vi "Read Number of peaks.vi"(8 "error in (no error)":errorcluster, 11 "Micron Optics Driver in":refnum<class "Micron Optics Driver.lvclass">) -> (0 "error out":errorcluster, 2 "Number of peaks":i32=4, 3 "Micron Optics Driver out":refnum<class "Micron Optics Driver.lvclass">)   [LabVIEW 2016, in "Micron Optics Driver.lvclass"]
uses:
  Micron Optics Driver.lvclass
  Micron Optics Driver.lvclass/Micron Optics Driver.ctl
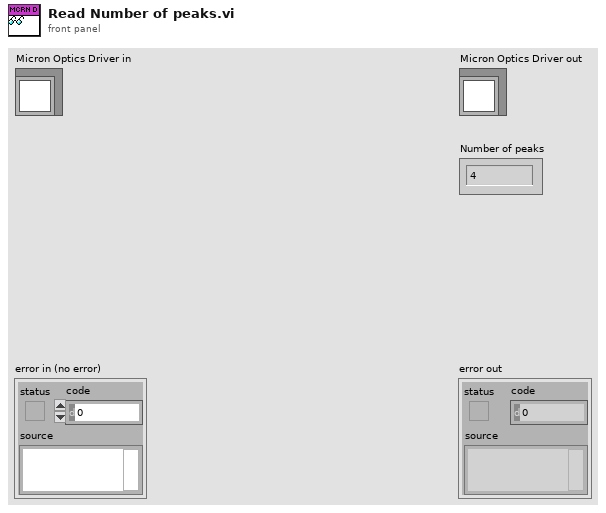
[diagram p1: front panel]
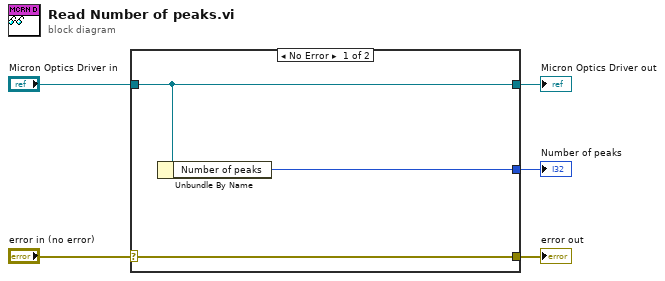
[diagram p0: block diagram]
diagram:
  n1 = case shown="No Error" "error in (no error)" {
    selector: "error in (no error)" -> [w8 w9]
    tunnel: [w8 w9] -> w4
    tunnel: [w7 w10] -> w2
    tunnel: "Micron Optics Driver in" -> [w7 w10]
    tunnel: [w6 _] -> w1
    frame No Error {
      n2 = Unbundle By Name(w7) -> ("Number of peaks"=w6:i32)
    }
    frame Error {
    }
  }
  "error out" <- w4
  "Micron Optics Driver out" <- w2
  "Number of peaks" <- w1
